vi "Triggered Acquisition.vi"(0 "RedPitaya TCP connection in":refnum<k5>, 2 "Trigger Mode":T1(ring), 4 "ms to wait trigger enable":u32, 5 "error in":errorcluster, 12 "timeout ms (2000)":i32=2000) -> (14 "RedPitaya TCP connection out":refnum<k5>, 19 "error out":errorcluster)   [LabVIEW 2021, in "RedPitaya.lvlib"]
doc: "Enables triggered data acquisition and sets the trigger mode."
uses:
  RedPitaya.lvlib
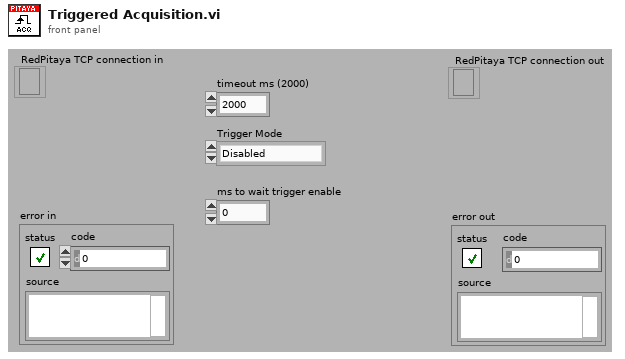
[diagram p1: front panel]
types:
  T1 = enum16{"Disabled", "Now", "Ch1 positive edge", "Ch1 negative edge", "Ch2 positive edge", "Ch2 negative edge", "external positive ege", "external negative edge", "AWG positive edge", "AWG negative edge"}
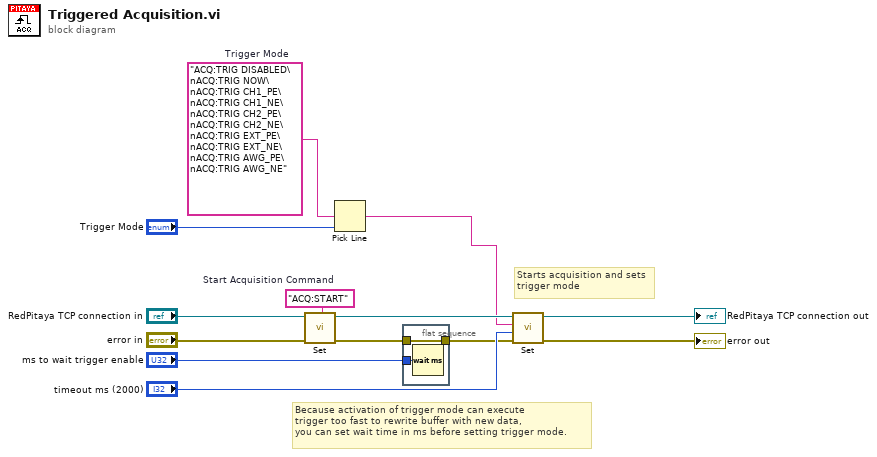
[diagram p0: block diagram]
diagram:
  w3 = "ACQ:TRIG DISABLED\nACQ:TRIG NOW\nACQ:TRIG CH1_PE\nACQ:TRIG CH1_NE\nACQ:TRIG CH2_PE\nACQ:TRIG CH2_NE\nACQ:TRIG EXT_PE\nACQ:TRIG EXT_NE\nACQ:TRIG AWG_PE\nACQ:TRIG AWG_NE"  # Trigger Mode
  w7 = "ACQ:START"  # Start Acquisition Command
  # "Because activation of trigger mode can execute\ntrigger too fast to rewrite buffer with new data,\nyou can set wait time in ms before setting trigger mode."
  # "Starts acquisition and sets\ntrigger mode"
  n1 = call "Set.vi"("error in"="error in", "SCPI Message"=w7, "RedPitaya connection in"="RedPitaya TCP connection in") -> ("error out"=w5:errorcluster, "RedPitaya connection out"=w9:refnum<k5>)  [unwired: 6 in, 1 out]
  n2 = Pick Line(multi-line string=w3, line index="Trigger Mode") -> (output string=w2:string)  [unwired: 1 in]
  n3 = flat-sequence {
    tunnel: "ms to wait trigger enable" -> [w15]
    tunnel: w5 -> [w14]
    tunnel: [w14] -> w4
    frame #0 {
      n4 = Wait (ms)(milliseconds to wait=w15) -> ()  [unwired: 1 out]
    }
  }
  n5 = call "Set.vi"("error in"=w4, "timeout ms (2000)"="timeout ms (2000)", "SCPI Message"=w2, "RedPitaya connection in"=w9) -> ("error out"=→"error out":errorcluster, "RedPitaya connection out"=→"RedPitaya TCP connection out":refnum<k5>)  [unwired: 5 in, 1 out]
